vi "myControlGUI.vi"() -> ()   [LabVIEW 2018]
panel:
  in  "取消按钮 2":bool
  in  "确定按钮 2":bool
  in  "终端滑模收敛时间":dbl(slide) scale=0.0..2.0
  in  "控制器参数α":dbl(slide) scale=0.0..100.0
  in  "控制器参数ε":dbl(slide) scale=0.0..1.0
  in  "控制器参数k":dbl(slide) scale=0.0..100.0
  in  "取消按钮":bool
  in  "确定按钮":bool
  in  "仿真启动":bool
  in  "控制器算法选择":string(combo)
  in  "终点相对惯性系z坐标":dbl
  in  "终点相对惯性系x坐标":dbl
  in  "终点相对惯性系y坐标":dbl
  in  "起点相对惯性系z坐标":dbl
  in  "起点相对惯性系x坐标":dbl
  in  "起点相对惯性系y坐标":dbl
  # "CRP14机械臂\n轨迹跟踪控制界面\n 杨海鑫毕业设计\n2016141442076"
  # "1.输入机械臂起点和终点位置，点击“确定坐标”按钮确认，点击“清除坐标”按钮将清除所有坐标数据；\n2.通过下拉栏选择控制算法，然后输入相应的控制器参数，点击“确定参数”按钮确认，点击“清除参数”按钮将清除参数数据；\n3.点击“仿真启动按钮“开始仿真。"
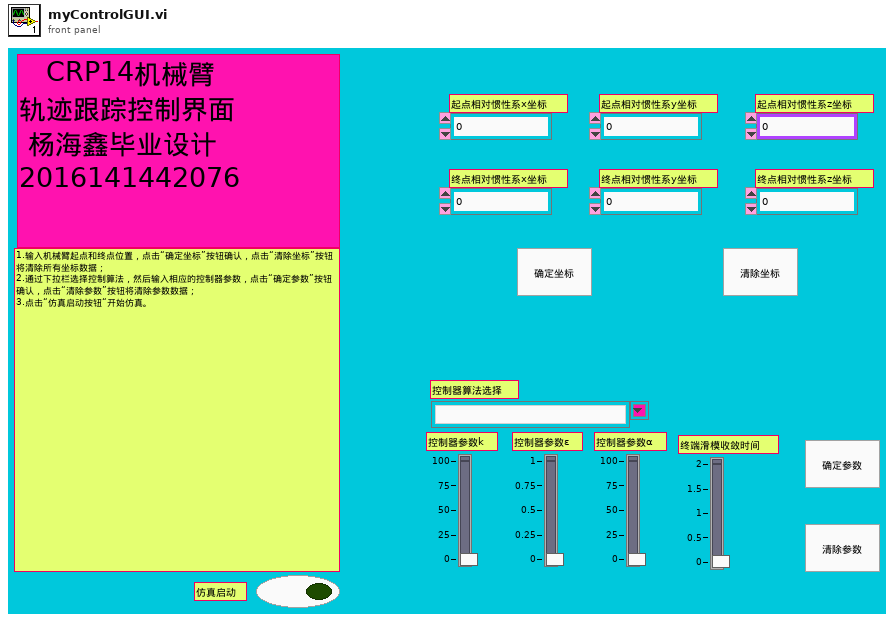
[diagram p1: front panel]
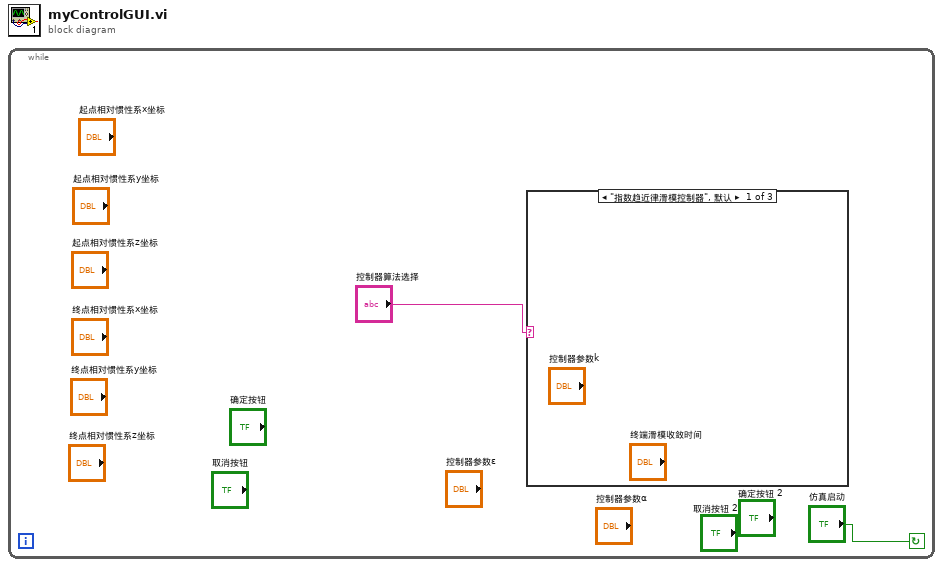
[diagram p0: block diagram]
diagram:
  n1 = while {
    stop <- "仿真启动" continue-if-true
    n2 = case shown="\"指数趋近律滑模控制器\", 默认" "控制器算法选择" {
      frame "指数趋近律滑模控制器", Default {
      }
      frame "改进趋近律滑模控制器" {
      }
      frame "有限时间终端滑模控制器" {
      }
    }
  }
